vi "Store Section Bounds Info.vi"(9 "Line Numbers":T1, 10 "Last row":i32) -> (3 "Section Data out":T3)   [LabVIEW 2018, in "Receipt Parsing.lvlib"]
uses:
  Receipt Parsing.lvlib
  Section Info--cluster.ctl
  Line Number.ctl
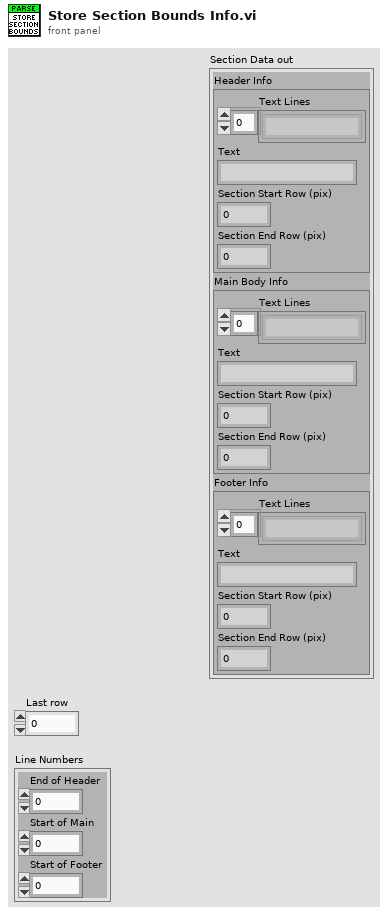
[diagram p1: front panel]
types:
  T1 = typedef "Receipt Parsing.lvlib/Line Number.ctl" = cluster{"End of Header":i32, "Start of Main":i32, "Start of Footer":i32}
  T2 = typedef "Receipt Parsing.lvlib/Section Info--cluster.ctl" = cluster{"Text Lines":string[], "Text":string, "Section Start Row (pix)":i32, "Section End Row (pix)":i32}
  T3 = cluster{"Header Info":T2, "Main Body Info":T2, "Footer Info":T2}
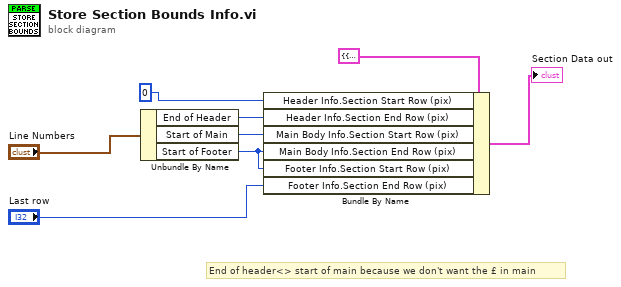
[diagram p0: block diagram]
diagram:
  # "End of header<> start of main because we don't want the £ in main"
  n1 = Unbundle By Name("Line Numbers") -> ("End of Header"=w5:i32, "Start of Main"=w6:i32, "Start of Footer"=w7:i32)
  n2 = Bundle By Name(cluster=T3 {"Header Info"={"Text Lines"=[], "Text"="", "Section Start Row (pix)"=0, "Section End Row (pix)"=0}, "Main Body Info"={"Text Lines"=[], "Text"="", "Section Start Row (pix)"=0, "Section End Row (pix)"=0}, "Footer Info"={"Text Lines"=[], "Text"="", "Section Start Row (pix)"=0, "Section End Row (pix)"=0}} ("Section Data out"), "Header Info.Section Start Row (pix)"=0, "Header Info.Section End Row (pix)"=w5, "Main Body Info.Section Start Row (pix)"=w6, "Main Body Info.Section End Row (pix)"=w7, "Footer Info.Section Start Row (pix)"=w7, "Footer Info.Section End Row (pix)"="Last row") -> (→"Section Data out":T3)
